vi "Back.vi"() -> ()   [LabVIEW 2021]
uses:
  TypeDef/Pin Levels Configuration.ctl
  TypeDef/Configure I2C Bus timing.ctl
  Demo_server/RPC Service/Communicate/Communicate.lvclass
  <vilib>/gRPC/LabVIEW gRPC Library/Shared/grpcId.ctl
  <vilib>/gRPC/LabVIEW gRPC Servicer/Servicer/Servicer.lvclass/Servicer.ctl
  Demo_server/RPC Service/Communicate/Communicate.lvclass/Communicate.ctl
  Demo_server/RPC Messages/Communication_ActionReply.ctl
  <vilib>/gRPC/LabVIEW gRPC Servicer/Servicer/Servicer.lvclass
  Demo_server/Demo_server.lvlib
  <vilib>/gRPC/LabVIEW gRPC Library/grpc-lvsupport-release.lvlib
panel:
  out "Configure I2C Bus timing":T1={"Frequency(Hz)"=10000.0, "T_HIGH(ns)"=0.0, "T_LOW(ns)"=0.0, "T_SU_STO(ns)"=0.0, "T_SU_STA(ns)"=0.0, "T_SU_DAT(ns)"=0.0, "T_BUF(ns)"=0.0, "T_HD_STA(ns)"=0.0, "T_HD_DAT(ns)"=0.0, "T.SU_ModSeIL(ns)"=40000.0, "T.HD_ModSeIL(ns)"=40000.0} {"T.HD_ModSeIL(ns)" min=40000.0 step=40000.0 format="%#_6p"; "T.SU_ModSeIL(ns)" min=40000.0 step=40000.0 format="%#_6p"; "Frequency(Hz)" min=10000.0 max=25000000.0 step=100.0 format="%#_6p"; "T_HD_DAT(ns)" step=1.0 format="%#_5g"; "T_SU_STA(ns)" min=0.0 step=1.0 format="%#_5g"; "T_HD_STA(ns)" min=0.0 step=1.0 format="%#_5g"; "T_SU_STO(ns)" min=0.0 step=1.0 format="%#_5g"; "T_BUF(ns)" min=0.0 step=1.0 format="%#_5g"; "T_HIGH(ns)" min=0.0 step=1.0 format="%#_5g"; "T_LOW(ns)" min=0.0 step=1.0 format="%#_5g"; "T_SU_DAT(ns)" step=1.0 format="%#_5g"}
  out "I2C Pin Levels":T2={"SCL VIH (V)"=0.0, "SCL VIL (V)"=0.0, "SCL Termination Mode"="Internal", "SCL Load Current (A)"=0.0015, "SDA VIH (V)"=0.0, "SDA VIL (V)"=0.0, "SDA Termination Mode"="Internal", "SDA Load Current (A)"=0.0015, "ModSeIL Termination Mode"="Internal", "ModSeIL VIL (V)"=0.0, "ModSeIL VIH (V)"=1.8} {"ModSeIL VIH (V)" min=-2.0 max=6.0 step=0.1 format="%#_2g"; "ModSeIL VIL (V)" min=-2.0 max=6.0 step=0.1 format="%#_2g"; "SDA Load Current (A)" min=0.0015 max=0.024 step=0.001 format="%#_2p"; "SDA VIH (V)" min=-2.0 max=6.0 step=0.1 format="%#_3g"; "SDA VIL (V)" min=-2.0 max=6.0 step=0.1 format="%#_3g"; "SCL Load Current (A)" min=0.0015 max=0.024 step=0.001 format="%#_2p"; "SCL VIH (V)" min=-2.0 max=6.0 step=0.1 format="%#_3g"; "SCL VIL (V)" min=-2.0 max=6.0 step=0.1 format="%#_3g"}
  out "Listening Port":i32
  # "Pin Levels Configuration"
  # "SCL"
  # "SDA"
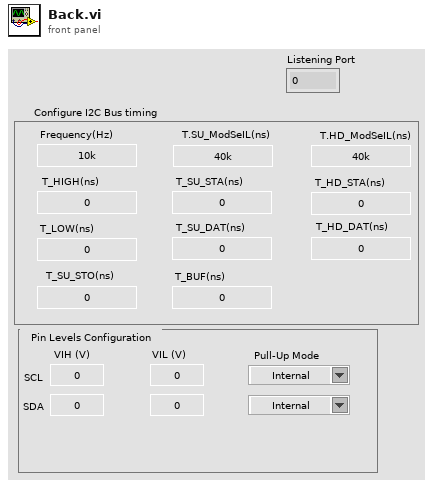
[diagram p1: front panel]
types:
  T1 = typedef "Configure I2C Bus timing.ctl" = cluster{"Frequency(Hz)":dbl, "T_HIGH(ns)":dbl, "T_LOW(ns)":dbl, "T_SU_STO(ns)":dbl, "T_SU_STA(ns)":dbl, "T_SU_DAT(ns)":dbl, "T_BUF(ns)":dbl, "T_HD_STA(ns)":dbl, "T_HD_DAT(ns)":dbl, "T.SU_ModSeIL(ns)":dbl, "T.HD_ModSeIL(ns)":dbl}
  T2 = typedef "Pin Levels Configuration.ctl" = cluster{"SCL VIH (V)":dbl, "SCL VIL (V)":dbl, "SCL Termination Mode":string, "SCL Load Current (A)":dbl, "SDA VIH (V)":dbl, "SDA VIL (V)":dbl, "SDA Termination Mode":string, "SDA Load Current (A)":dbl, "ModSeIL Termination Mode":string, "ModSeIL VIL (V)":dbl, "ModSeIL VIH (V)":dbl}
  T3 = typedef "grpc-lvsupport-release.lvlib/grpcId.ctl" = u64
  T4 = typedef "Demo_server.lvlib/Communicate.lvclass/Server gRPC UEs.ctl" = cluster{"Communicate Transmission gRPC UE":refnum<user-event>}
  T5 = typedef "Demo_server.lvlib/Communication_ActionReply.ctl" = cluster{"Reply":string, "Status":string}
  T6 = typedef "Demo_server.lvlib/Communication_ActionRequest.ctl" = cluster{"Request":string, "Data":string}
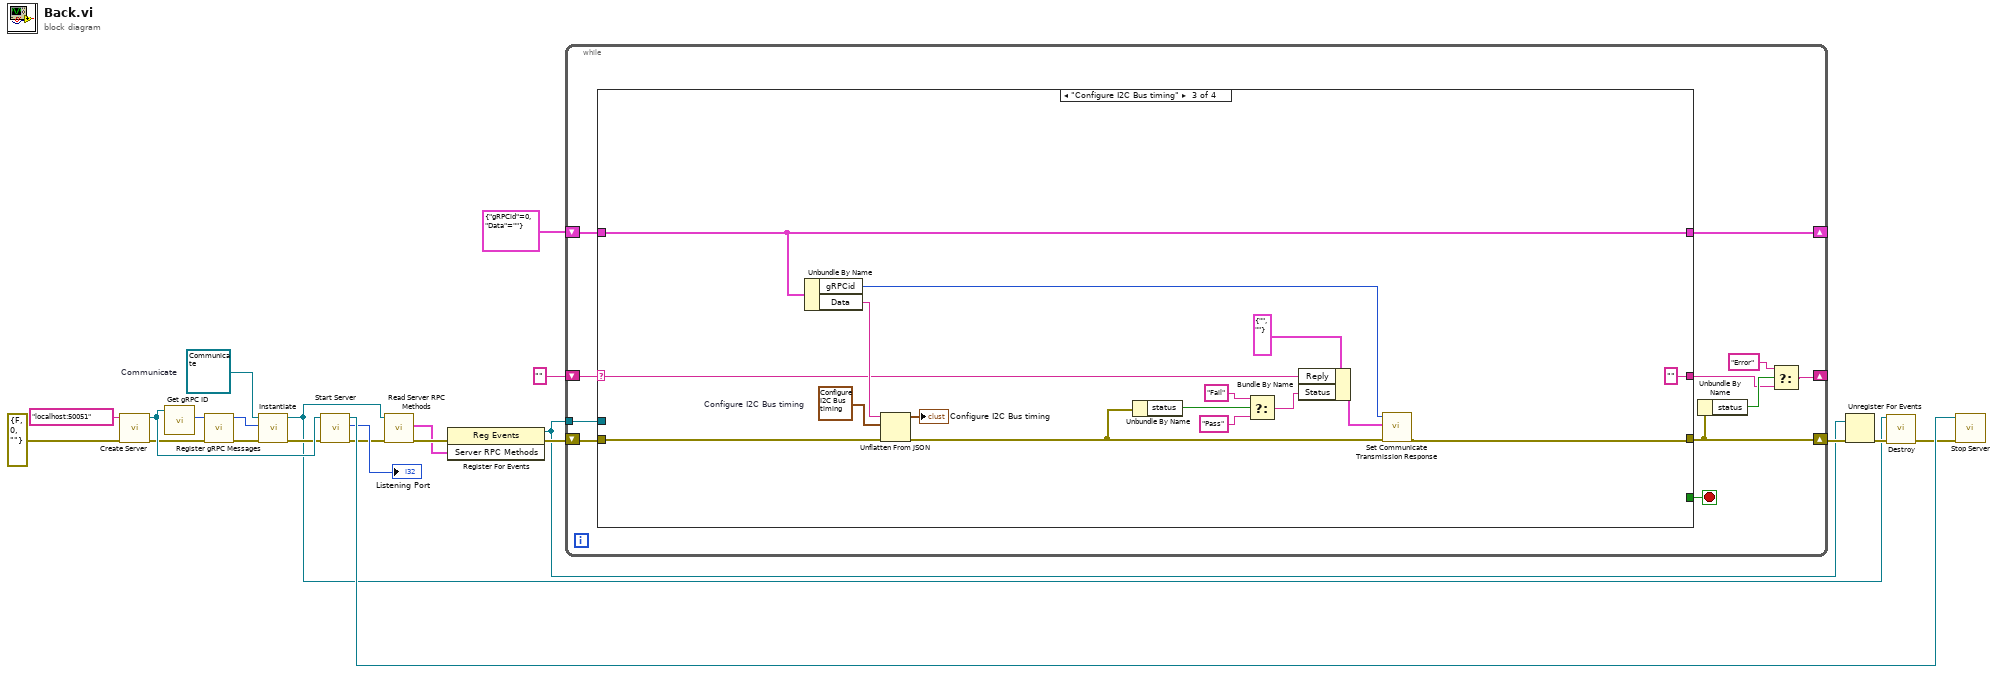
[diagram p0: block diagram]
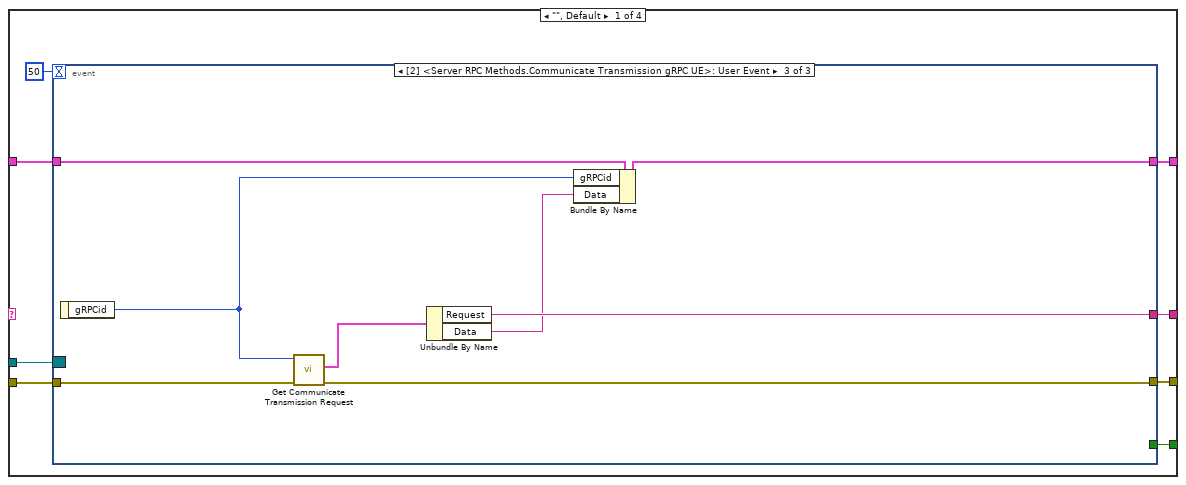
[diagram p2: hidden frame]
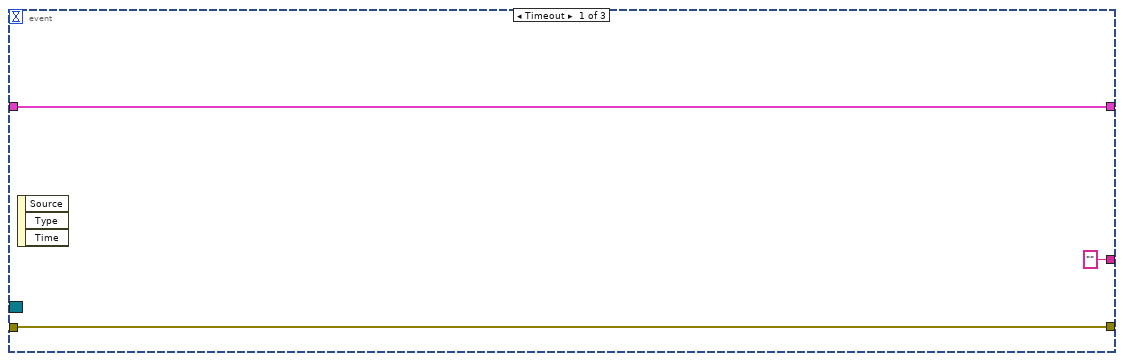
[diagram p3: hidden frame]
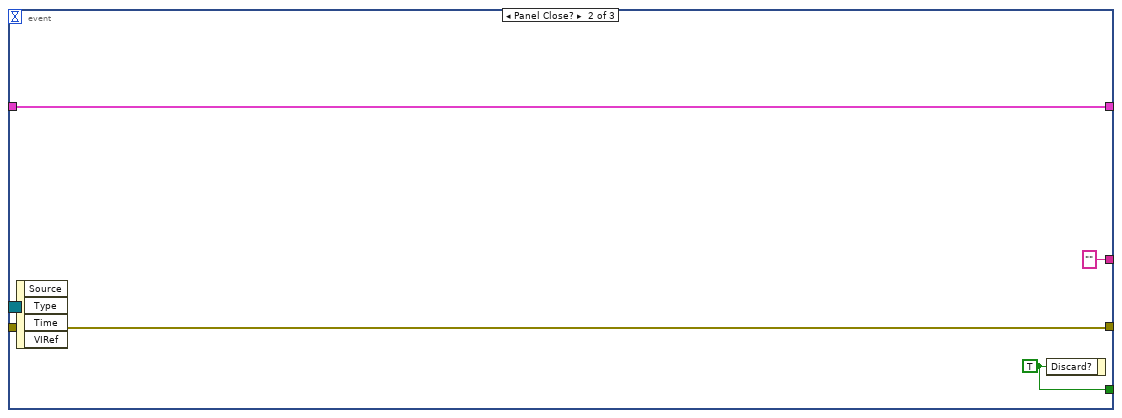
[diagram p4: hidden frame]
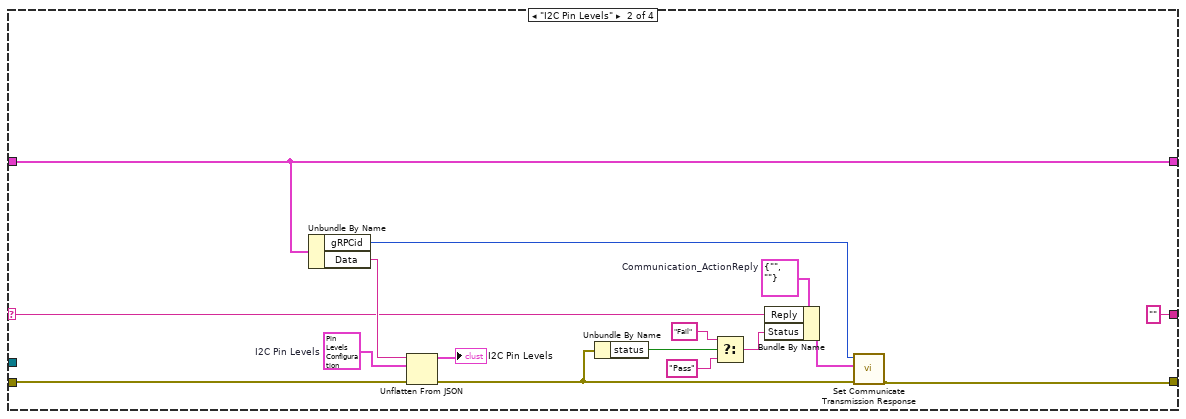
[diagram p5: hidden frame]
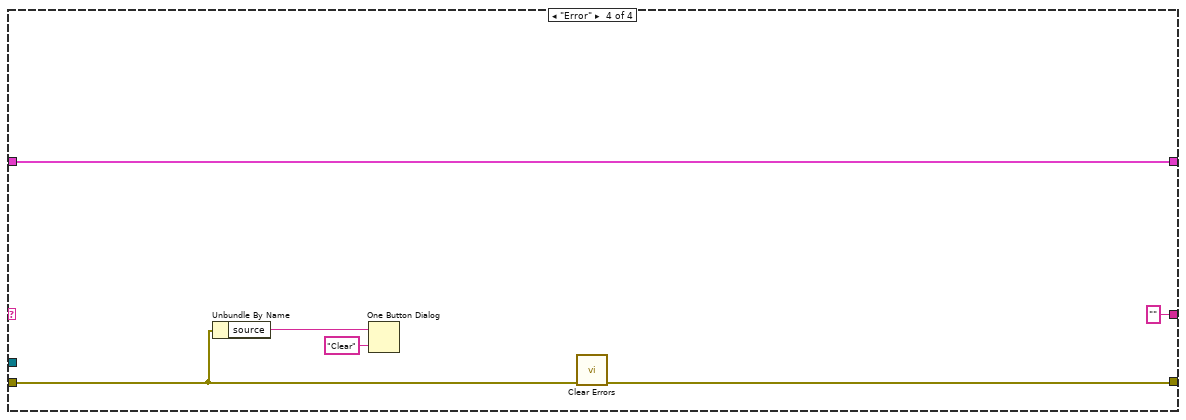
[diagram p6: hidden frame]
diagram:
  w10 = refnum<class "Communicate.lvclass"> refnum  # Communicate
  n1 = call <vilib>:"Create Server.vi"("error in"=errorcluster {"status"=FALSE, "code"=0, "source"=""} ("error in (no error)"), "Server Address"="localhost:50051") -> ("error out"=w3:errorcluster, "gRPC Server out"=w14:refnum<class "Servicer.lvclass">)  [unwired: 8 in]
  n2 = call <vilib>:"Get gRPC ID.vi"("OOP Server in"=w14) -> ("gRPC ID"=w4:T3)  [unwired: 9 in, 1 out]
  n3 = call "Register gRPC Messages.vi"("error in (no error)"=w3, "gRPC ID"=w4) -> ("error out"=w2:errorcluster, "gRPC ID Out"=w5:T3)  [unwired: 8 in]
  n4 = call-dynamic "Instantiate.vi"("error in"=w2, "gRPCid"=w5, "iService"=w10) -> ("error out"=w13:errorcluster, "iService"=w7:refnum<class "Communicate.lvclass">)  [unwired: 7 in]
  n5 = call <vilib>:"Start Server.vi"("error in"=w13, "gRPC Server in"=w14) -> ("error out"=w6:errorcluster, "Listening Port"=→"Listening Port":i32, "gRPC Server out"=w16:refnum<class "Servicer.lvclass">)  [unwired: 7 in]
  n6 = call "Read Server RPC Methods.vi"("error in (no error)"=w6, "SignalGeneratorService in"=w7) -> ("error out"=w9:errorcluster, "Server RPC Methods"=w8:T4)  [unwired: 7 in, 1 out]
  n7 = register-events(error in=w9, w8) -> (reference out=w19:refnum<event-registration>, error out=w21:errorcluster)  [unwired: 1 in]
  n8 = while {
    shift-right: [w30] -> w20
    shift-left: w21 -> [w32]
    shift-right: [w28] -> _
    shift-left: "" -> [w33]
    tunnel: w19 -> [w25]
    shift-right: [w24] -> _
    shift-left: cluster{"gRPCid":T3, "Data":string} {"gRPCid"=0, "Data"=""} -> [w23]
    stop <- w31 stop-if-true
    n9 = case shown="\"Configure I2C Bus timing\"" w33 {
      selector: w33 -> [_ w64 w81 _]
      tunnel: w32 -> [w41 w70 w86 w93]
      tunnel: [w40 w72 w88 w94] -> w30
      tunnel: [w39 "" ("Request") "" ("Request") ""] -> w27
      tunnel: [w38 _ _ _] -> w31
      tunnel: w25 -> [w36 _ _ _]
      tunnel: [w35 w71 w87 w89] -> w24
      tunnel: w23 -> [w34 w71 w87 w89]
      frame "", Default {
        n10 = event shown="[2] <Server RPC Methods.Communicate Transmission gRPC UE>: User Event" {
          selector: w36 -> [_ _ _]
          dyn-events: _ -> [_ _ _]
          timeout: 50 -> [_ _ _]
          tunnel: w41 -> [w44 w48 w56]
          tunnel: [w44 w48 w49] -> w40
          tunnel: ["" "" w54] -> w39
          tunnel: [_ w46 _] -> w38
          tunnel: [w42 w45 w52] -> w35
          tunnel: w34 -> [w42 w45 w53]
          event Timeout {
            n11 = event-data() -> ()  [unwired: 1 in, 3 out]
          }
          event Panel Close? {
            w46 = TRUE ("Discard?")
            n12 = event-data() -> ()  [unwired: 1 in, 4 out]
            n13 = event-data("Discard?"=w46) -> ()  [unwired: 1 in, 1 out]
          }
          event User Event {
            n14 = event-data() -> ("gRPCid"=w51:T3)  [unwired: 1 in]
            n15 = call "Get Communicate Transmission Request.vi"("error in (no error)"=w56, "gRPCid in"=w51) -> ("error out"=w49:errorcluster, "Message Data"=w55:T6)  [unwired: 7 in, 1 out]
            n16 = Unbundle By Name(w55) -> ("Request"=w54:string, "Data"=w50:string)
            n17 = Bundle By Name(cluster=w53, "gRPCid"=w51, "Data"=w50) -> (w52:cluster{"gRPCid":T3, "Data":string})
          }
        }
      }
      frame "I2C Pin Levels" {
        w66 = T5 {"Reply"="", "Status"=""}  # Communication_ActionReply
        w68 = T2 {"SCL VIH (V)"=0.0, "SCL VIL (V)"=0.0, "SCL Termination Mode"="Internal", "SCL Load Current (A)"=0.0015, "SDA VIH (V)"=0.0, "SDA VIL (V)"=0.0, "SDA Termination Mode"="Internal", "SDA Load Current (A)"=0.0015, "ModSeIL Termination Mode"="Internal", "ModSeIL VIL (V)"=0.0, "ModSeIL VIH (V)"=1.8}  # I2C Pin Levels
        n18 = Unbundle By Name(w71) -> ("gRPCid"=w57:T3, "Data"=w69:string)
        n19 = Unflatten From JSON(JSON string=w69, type and defaults=w68, error in (no error)=w70) -> (value=→"I2C Pin Levels":T2, error out=w60:errorcluster)  [unwired: 4 in]
        n20 = Unbundle By Name(w60) -> ("status"=w59:bool)
        n21 = Select(t="Fail", s=w59, f="Pass" ("Status")) -> (s? t:f=w63:string)
        n22 = Bundle By Name(cluster=w66, "Reply"=w64, "Status"=w63) -> (w65:T5)
        n23 = call "Set Communicate Transmission Response.vi"("error in (no error)"=w60, "Message Data"=w65, "gRPCid in"=w57) -> ("error out"=w72:errorcluster)  [unwired: 8 in]
      }
      frame "Configure I2C Bus timing" {
        w74 = T1 {"Frequency(Hz)"=10000.0, "T_HIGH(ns)"=0.0, "T_LOW(ns)"=0.0, "T_SU_STO(ns)"=0.0, "T_SU_STA(ns)"=0.0, "T_SU_DAT(ns)"=0.0, "T_BUF(ns)"=0.0, "T_HD_STA(ns)"=0.0, "T_HD_DAT(ns)"=0.0, "T.SU_ModSeIL(ns)"=40000.0, "T.HD_ModSeIL(ns)"=40000.0}  # Configure I2C Bus timing
        n24 = Unbundle By Name(w87) -> ("gRPCid"=w75:T3, "Data"=w85:string)
        n25 = Unflatten From JSON(JSON string=w85, type and defaults=w74, error in (no error)=w86) -> (value=→"Configure I2C Bus timing":T1, error out=w77:errorcluster)  [unwired: 4 in]
        n26 = Unbundle By Name(w77) -> ("status"=w76:bool)
        n27 = Select(t="Fail", s=w76, f="Pass" ("Status")) -> (s? t:f=w80:string)
        n28 = Bundle By Name(cluster=T5 {"Reply"="", "Status"=""} ("Message Data"), "Reply"=w81, "Status"=w80) -> (w82:T5)
        n29 = call "Set Communicate Transmission Response.vi"("error in (no error)"=w77, "Message Data"=w82, "gRPCid in"=w75) -> ("error out"=w88:errorcluster)  [unwired: 8 in]
      }
      frame "Error" {
        n30 = Unbundle By Name(w93) -> ("source"=w91:string)
        n31 = One Button Dialog(message=w91, button name ("OK")="Clear") -> ()  [unwired: 1 out]
        n32 = call <vilib>:"Clear Errors.vi"("error in (no error)"=w93) -> ("error out"=w94:errorcluster)  [unwired: 5 in, 1 out]
      }
    }
    n33 = Unbundle By Name(w30) -> ("status"=w29:bool)
    n34 = Select(t="Error", s=w29, f=w27) -> (s? t:f=w28:string)
  }
  n35 = Unregister For Events(event registration refnum=w19, error in=w20) -> (error out=w11:errorcluster)
  n36 = call-dynamic "Destroy.vi"("error in (no error)"=w11, "SignalGeneratorService in"=w7) -> ("error out"=w12:errorcluster)  [unwired: 8 in, 1 out]
  n37 = call <vilib>:"Stop Server.vi"("error in"=w12, "gRPC Server in"=w16) -> ()  [unwired: 9 in, 1 out]
